vi "OpenDataFIle.vi"(11 "Data":string) -> ()   [LabVIEW 2019]
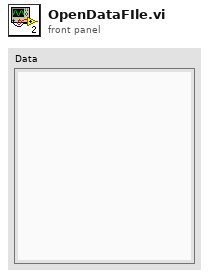
[diagram p1: front panel]
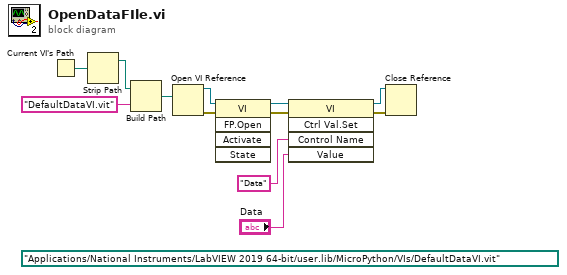
[diagram p0: block diagram]
diagram:
  (unwired) path "/Applications/National Instruments/LabVIEW 2019 64-bit/user.lib/MicroPython/VIs/DefaultDataVI.vit" ("vi path")
  n1 = Current VI's Path() -> (path=w4:path)
  n2 = Strip Path(path=w4) -> (stripped path=w3:path)  [unwired: 1 out]
  n3 = Build Path(base path=w3, name or relative path="DefaultDataVI.vit") -> (appended path=w1:path)
  n4 = Open VI Reference(vi path=w1) -> (vi reference=w12:refnum<vi>, error out=w11:errorcluster)  [unwired: 5 in]
  n5 = invoke class="VI" method="FP.Open"(reference=w12, error in=w11) -> (reference out=w8:refnum<vi>, error out=w7:errorcluster)  [unwired: 3 in, 3 out]
  n6 = invoke class="VI" method="Ctrl Val.Set"(reference=w8, error in=w7, "Control Name"="Data", "Value"="Data") -> (reference out=w6:refnum<vi>, error out=w5:errorcluster)  [unwired: 1 in, 3 out]
  n7 = Close Reference(reference=w6, error in (no error)=w5) -> ()  [unwired: 1 out]
